vi "Trends.vi"() -> ()   [LabVIEW 2018]
panel:
  in  "Enable Level 3":bool
  in  "Enable Level 2":bool
  in  "Enable Level":bool
  in  "Pressure Unit":enum16{"Bar", "kPascal", "PSI"}(ring)
  in  "Temperature unit":enum16{"Celsius", "Farenheit", "Kelvin"}(ring)
  in  "Level unit:":enum16{"Level", "Volume", "Percentage"}(ring)
  in  "Tab Control":T1(tab)
  out "Tank 1 Trends":cluster{"X":dbl, "Y":dbl}[](graph)
  out "Tank 1 Trends 2":cluster{"X":dbl, "Y":dbl}[](graph)
  out "Tank 1 Trends 3":cluster{"X":dbl, "Y":dbl}[](graph)
  out "Tank 1 Trends 4":cluster{"X":dbl, "Y":dbl}[](graph)
  in  "stop":bool
  # "Display Options"
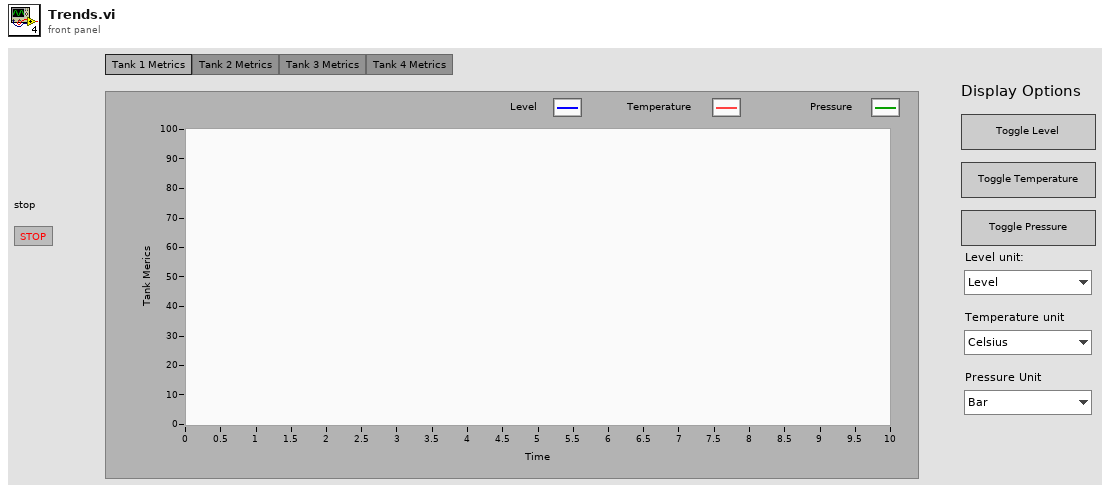
[diagram p1: front panel]
types:
  T1 = enum32{"Tank 1 Metrics", "Tank 2 Metrics", "Tank 3 Metrics", "Tank 4 Metrics"}
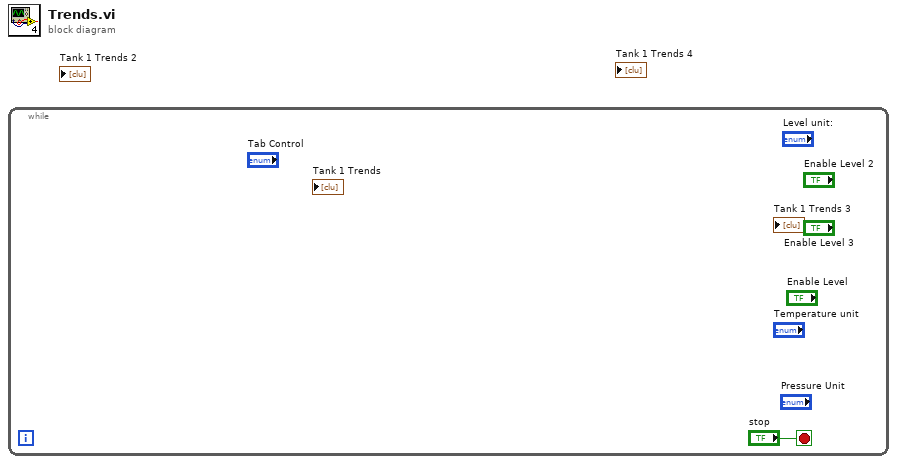
[diagram p0: block diagram]
diagram:
  n1 = while {
    stop <- "stop" stop-if-true
  }
